vi "calculate_percentage_compression.vi"(9 "compression bit length":i32[](array[numeric]), 11 "original bit length":i32[](array[numeric])) -> (3 "percentage compression":i32)   [LabVIEW 2018]
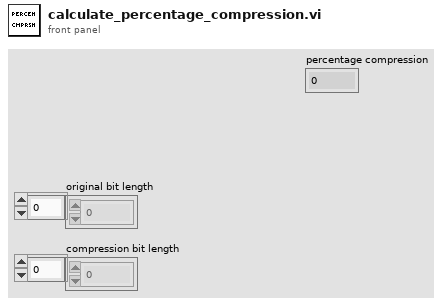
[diagram p1: front panel]
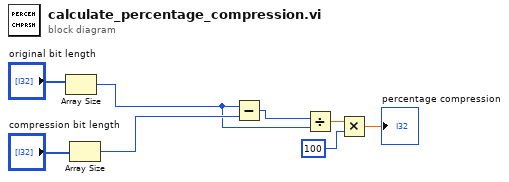
[diagram p0: block diagram]
diagram:
  n1 = Array Size(array="original bit length") -> (size(s)=w1:i32)
  n2 = Array Size(array="compression bit length") -> (size(s)=w2:i32)
  n3 = Subtract(x=w1, y=w2) -> (x-y=w8:i32)
  n4 = Divide(x=w8, y=w1) -> (x/y=w7:dbl)
  n5 = Multiply(x=w7, y=100) -> (x*y=→"percentage compression":dbl)
